vi "Field jsObject.vi"(8 "error in (no error)":errorcluster, 9 "Field Record (empty)":T1={"ixField"=0, "iSequenceOrder"=0, "sxFieldId"="", "sxSequenceId"="", "sDisplayName"="", "sValue"="", "sUnits"="", "nDataType"=enum."timestamp", "nNextItem"=enum."Reset", "fSystem"=FALSE, "fSystemValue"=FALSE, "fRequired"=FALSE, "fSetAtTest"=FALSE, "fTestField"=FALSE, "fDeleted"=FALSE, "fIndexed"=FALSE, "fFreeList"=FALSE}, 10 "Field jsObject Name (\"\")":string, 11 "Previous String (\"\")":string) -> (0 "error out":errorcluster, 2 "Field jsObject":string, 3 "Field jsObject Definition":string)   [LabVIEW 2011]
uses:
  Field Record.ctl
  Field DataTypes.ctl
  Field NextItem.ctl
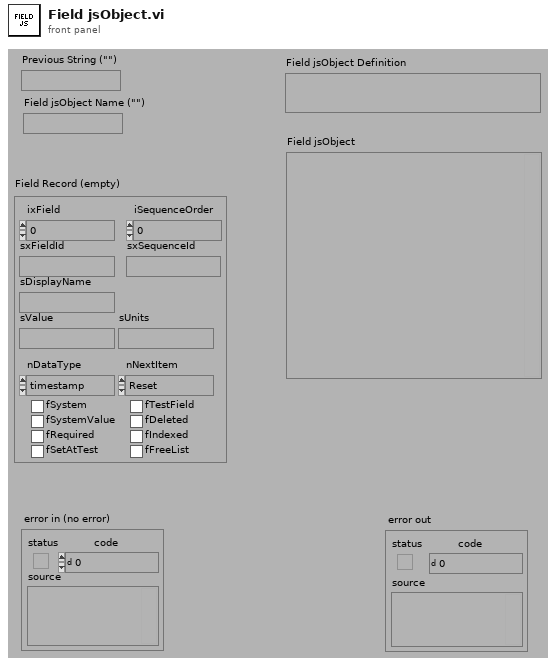
[diagram p1: front panel]
types:
  T1 = typedef "Field Record.ctl" = cluster{"ixField":i32, "iSequenceOrder":i32, "sxFieldId":string, "sxSequenceId":string, "sDisplayName":string, "sValue":string, "sUnits":string, "nDataType":T2, "nNextItem":T3, "fSystem":bool, "fSystemValue":bool, "fRequired":bool, "fSetAtTest":bool, "fTestField":bool, "fDeleted":bool, "fIndexed":bool, "fFreeList":bool}
  T2 = typedef "Field DataTypes.ctl" = enum32{"text", "numeric", "list", "timestamp", "boolean"}
  T3 = typedef "Field NextItem.ctl" = enum32{"Reset", "Retain", "Auto-Increment"}
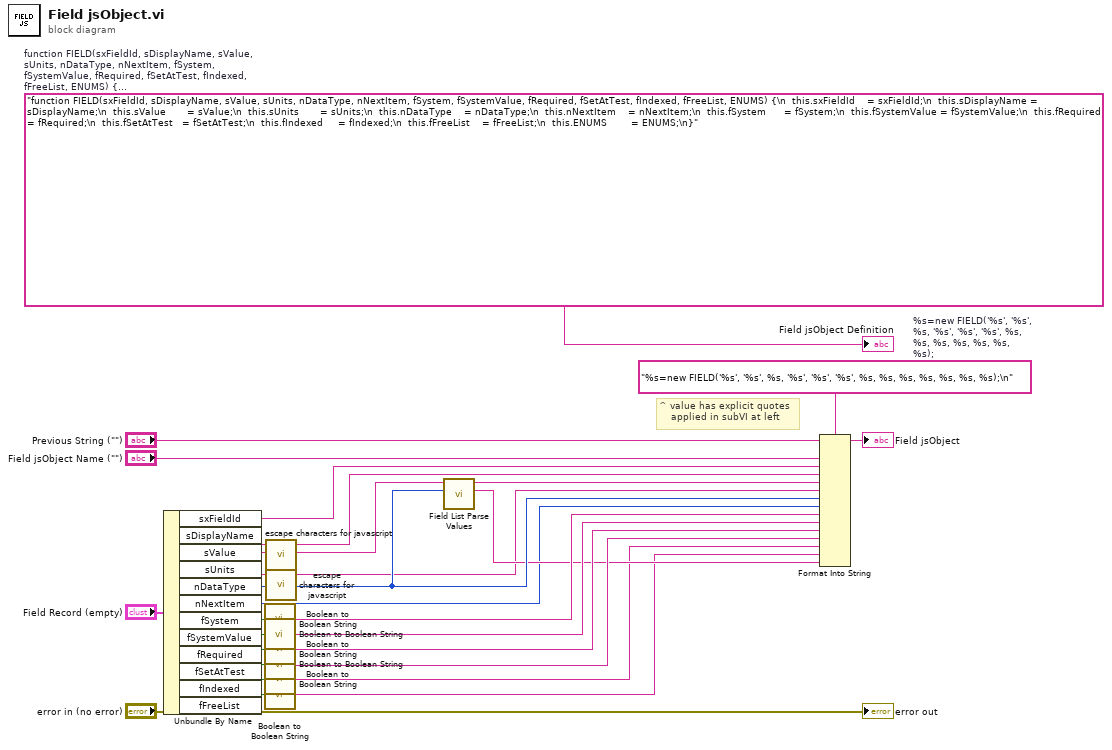
[diagram p0: block diagram]
diagram:
  w14 = "function FIELD(sxFieldId, sDisplayName, sValue, sUnits, nDataType, nNextItem, fSystem, fSystemValue, fRequired, fSetAtTest, fIndexed, fFreeList, ENUMS) {\n  this.sxFieldId    = sxFieldId;\n  this.sDisplayName = sDisplayName;\n  this.sValue       = sValue;\n  this.sUnits       = sUnits;\n  this.nDataType    = nDataType;\n  this.nNextItem    = nNextItem;\n  this.fSystem      = fSystem;\n  this.fSystemValue = fSystemValue;\n  this.fRequired    = fRequired;\n  this.fSetAtTest   = fSetAtTest;\n  this.fIndexed     = fIndexed;\n  this.fFreeList    = fFreeList;\n  this.ENUMS        = ENUMS;\n}"  # function FIELD(sxFieldId, sDisplayName, sValue, sUnits, nDataType, nNextItem, fSystem, fSystemValue, fRequired, fSetAtTest, fIndexed, fFreeList, ENUMS) {   this.sxFieldId    = sxFieldId;   this.sDisplayName = sDisplayName;   this.sValue       = sValue;   this.sUnits       = sUnits;   this.nDataType    = nDataType;   this.nNextItem    = nNextItem;   this.fSystem      = fSystem;   this.fSystemValue = fSystemValue;   this.fRequired    = fRequired;   this.fSetAtTest   = fSetAtTest;   this.fIndexed     = fIndexed;   this.fFreeList    = fFreeList;   this.ENUMS        = ENUMS; }
  w29 = "%s=new FIELD('%s', '%s', %s, '%s', '%s', '%s', %s, %s, %s, %s, %s, %s, %s);\n"  # %s=new FIELD('%s', '%s', %s, '%s', '%s', '%s', %s, %s, %s, %s, %s, %s, %s);
  # "^ value has explicit quotes\n    applied in subVI at left"
  n1 = Unbundle By Name("Field Record (empty)") -> ("sxFieldId"=w21:string, "sDisplayName"=w11:string, "sValue"=w1:string, "sUnits"=w9:string, "nDataType"=w15:T2, "nNextItem"=w7:T3, "fSystem"=w19:bool, "fSystemValue"=w18:bool, "fRequired"=w17:bool, "fSetAtTest"=w16:bool, "fIndexed"=w6:bool, "fFreeList"=w4:bool)
  n2 = call "Boolean to Boolean String.vi"("Boolean"=w19) -> ("Boolean string"=w25:string)  [unwired: 1 in]
  n3 = call "Boolean to Boolean String.vi"("Boolean"=w18) -> ("Boolean string"=w28:string)  [unwired: 1 in]
  n4 = call "Boolean to Boolean String.vi"("Boolean"=w17) -> ("Boolean string"=w27:string)  [unwired: 1 in]
  n5 = call "Boolean to Boolean String.vi"("Boolean"=w16) -> ("Boolean string"=w26:string)  [unwired: 1 in]
  n6 = call "Boolean to Boolean String.vi"("Boolean"=w6) -> ("Boolean string"=w5:string)  [unwired: 1 in]
  n7 = call "Boolean to Boolean String.vi"("Boolean"=w4) -> ("Boolean string"=w3:string)  [unwired: 1 in]
  n8 = call "escape characters for javascript.vi"("String (\"\")"=w11) -> ("escaped String"=w10:string)  [unwired: 4 out]
  n9 = call "escape characters for javascript.vi"("String (\"\")"=w9) -> ("escaped String"=w8:string)  [unwired: 4 out]
  n10 = call "Field List Parse Values.vi"("nDataType"=w15, "sValue"=w1) -> ("js List Array"=w13:string, "Current Value"=w2:string)  [unwired: 1 in, 7 out]
  n11 = Format Into String(format string=w29, initial string="Previous String (\"\")", "Field jsObject Name (\"\")", w21, w10, w2, w8, w15, w7, w25, w28, w27, w26, w5, w3, w13) -> (resulting string=→"Field jsObject":string)  [unwired: 1 in, 1 out]
  "error out" <- "error in (no error)"
  "Field jsObject Definition" <- w14
